vi "Append Table.vi"(8 "error in (no error)":errorcluster, 9 "Table Style":refnum<class "Style.lvclass">, 10 "Table":string[][](array[string]), 11 "xwpfWriter in":refnum<class "xwpfWriter.lvclass">) -> (0 "error out":errorcluster, 3 "xwpfWriter out":refnum<class "xwpfWriter.lvclass">)   [LabVIEW 2017, in "LabVIEW NPOI.lvlib" / "xwpfWriter.lvclass"]
uses:
  xwpfWriter.lvclass
  Styles/Style/Style.lvclass
  xwpfWriter.lvclass/xwpfWriter.ctl
  C:/Users/Neo/Desktop/Dev_Tools_BR/LabVIEW_NPOI/lib/NPOI 2.1.1/NPOI.OOXML.dll
  lib/NPOI 2.1.1/NPOI.OOXML.dll
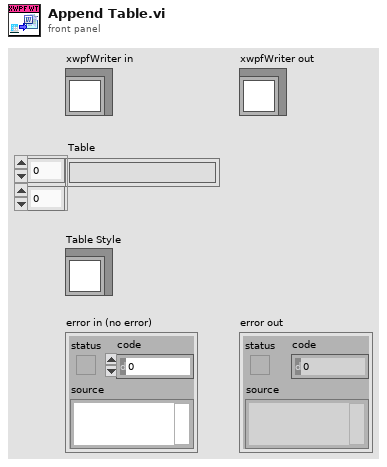
[diagram p1: front panel]
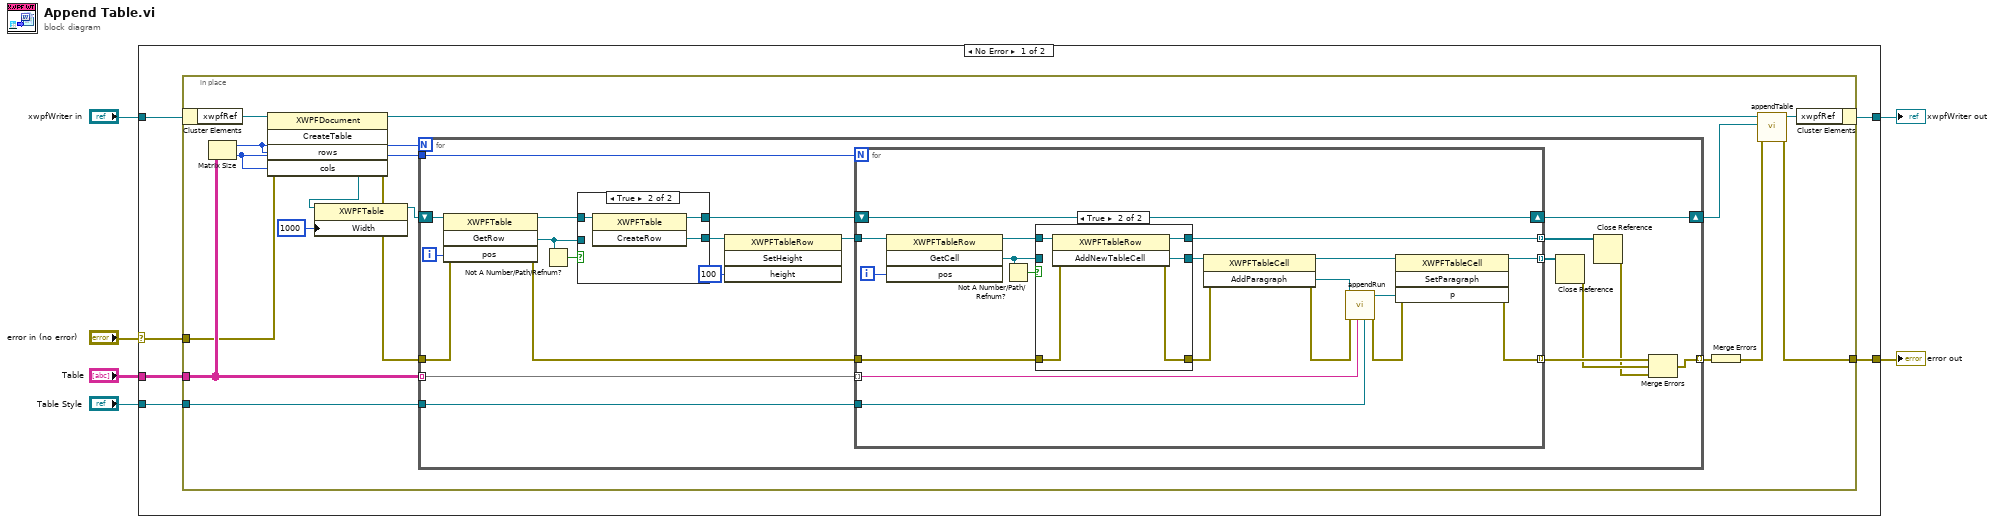
[diagram p0: block diagram]
diagram:
  n1 = case shown="No Error" "error in (no error)" {
    selector: "error in (no error)" -> [w10 w82]
    tunnel: [w8 w82] -> w5
    tunnel: [w12 w81] -> w3
    tunnel: "xwpfWriter in" -> [w11 w81]
    tunnel: "Table" -> [w9 _]
    tunnel: "Table Style" -> [w7 _]
    frame No Error {
      n2 = in-place {
        in-place-border: w10 -> [w26]
        in-place-border: w9 -> [w27]
        in-place-border: [w20] -> w8
        in-place-border: w7 -> [w13]
        n3 = in-place-cluster #1(w11) -> ("xwpfRef"=w28:refnum<k24>)
        n4 = Matrix Size(0:w27) -> (1:w16:i32, 2:w15:i32)
        n5 = invoke class="XWPFDocument" method="CreateTable"(reference=w28, error in=w26, "rows"=w16, "cols"=w15) -> (reference out=w17:refnum<k24>, error out=w25:errorcluster, "CreateTable"=w14:refnum<k24>)  [unwired: 1 in, 2 out]
        n6 = property class="XWPFTable"(reference=w14, "Width"=1000) -> (reference out=w18:refnum<k24>)  [unwired: 1 in, 1 out]
        n7 = for {
          N: w16 -> [_]
          tunnel: w15 -> [w48]
          tunnel: w27 -> [w47] mode=indexing
          tunnel: w25 -> [w45]
          tunnel: [w38] -> w24 mode=indexing
          shift-right: [w43] -> w22
          shift-left: w18 -> [w49]
          tunnel: w13 -> [w29]
          i -> [w31]
          n8 = invoke class="XWPFTable" method="GetRow"(reference=w49, error in=w45, "pos"=w31) -> (reference out=w37:refnum<k24>, error out=w44:errorcluster, "GetRow"=w35:refnum<k24>)  [unwired: 1 in, 1 out]
          n9 = Not A Number/Path/Refnum?(number/path/refnum=w35) -> (NaN/Path/Refnum?=w36:bool)
          n10 = case shown="True" w36 {
            tunnel: w37 -> [w51 w54]
            tunnel: [w51 w53] -> w32
            tunnel: [w50 w52] -> w34
            tunnel: w35 -> [w50 _]
            frame False {
            }
            frame True {
              n11 = invoke class="XWPFTable" method="CreateRow"(reference=w54) -> (reference out=w53:refnum<k24>, "CreateRow"=w52:refnum<k24>)  [unwired: 2 in, 1 out]
            }
          }
          n12 = invoke class="XWPFTableRow" method="SetHeight"(reference=w34, "height"=100) -> (reference out=w33:refnum<k24>)  [unwired: 2 in, 3 out]
          n13 = for {
            N: w48 -> [_]
            tunnel: w47 -> [w56] mode=indexing
            tunnel: [w64] -> w42 mode=indexing
            tunnel: w44 -> [w70]
            tunnel: [w57] -> w46 mode=indexing
            shift-right: [w71] -> w43
            shift-left: w32 -> [w71]
            tunnel: [w72] -> w41 mode=indexing
            tunnel: w33 -> [w69]
            tunnel: w29 -> [w55]
            i -> [w67]
            n14 = invoke class="XWPFTableRow" method="GetCell"(reference=w69, "pos"=w67) -> (reference out=w68:refnum<k24>, "GetCell"=w66:refnum<k24>)  [unwired: 2 in, 2 out]
            n15 = Not A Number/Path/Refnum?(number/path/refnum=w66) -> (NaN/Path/Refnum?=w65:bool)
            n16 = case shown="True" w65 {
              tunnel: [w75 w80] -> w63
              tunnel: [w73 w79] -> w60
              tunnel: [w74 w78] -> w72
              tunnel: w70 -> [w73 w77]
              tunnel: w68 -> [w74 w76]
              tunnel: w66 -> [w75 _]
              frame False {
              }
              frame True {
                n17 = invoke class="XWPFTableRow" method="AddNewTableCell"(reference=w76, error in=w77) -> (reference out=w78:refnum<k24>, error out=w79:errorcluster, "AddNewTableCell"=w80:refnum<k24>)  [unwired: 1 in]
              }
            }
            n18 = invoke class="XWPFTableCell" method="AddParagraph"(reference=w63, error in=w60) -> (error out=w59:errorcluster, "AddParagraph"=w62:refnum<k24>)  [unwired: 1 in, 1 out]
            n19 = call "appendRun.vi"("Style"=w55, "value"=w56, "error in (no error)"=w59, "Paragraph in"=w62) -> ("error out"=w58:errorcluster, "reference out"=w61:refnum<k24>)  [unwired: 6 in]
            n20 = invoke class="XWPFTableCell" method="SetParagraph"(reference=w63, error in=w58, "p"=w61) -> (reference out=w64:refnum<k24>, error out=w57:errorcluster)  [unwired: 1 in, 2 out]
          }
          n21 = Close Reference(reference=w42) -> (error out=w40:errorcluster)  [unwired: 1 in]
          n22 = Close Reference(reference=w41) -> (error out=w39:errorcluster)  [unwired: 1 in]
          n23 = Merge Errors(w46, w40, w39) -> (w38:errorcluster)
        }
        n24 = Merge Errors(w24) -> (w21:errorcluster)
        n25 = call "appendTable.vi"("error in (no error)"=w21, "table"=w22, "XWPFDocuement in"=w17) -> ("error out"=w20:errorcluster, "XWPFDocuement out"=w23:refnum<k24>)  [unwired: 7 in]
        n26 = in-place-cluster #1("xwpfRef"=w23) -> (w12:refnum<class "xwpfWriter.lvclass">)
      }
    }
    frame Error {
    }
  }
  "error out" <- w5
  "xwpfWriter out" <- w3
